vi "SutterController.vi"() -> ()   [LabVIEW 2014]
uses:
  SerialController/Serial Controller.lvclass
  GlobalVars.vi
  <vilib>/Analysis/Matrix/Numeric/Conversions/Array To Matrix - RA2.vi
  <vilib>/Analysis/Matrix/Numeric/Conversions/Array To Matrix - RA.vi
  <vilib>/Analysis/Matrix/Numeric/Multiply/Multiply - RM,RM.vi
  <vilib>/Analysis/Matrix/Numeric/Conversions/Matrix To Array - RM.vi
  <vilib>/Analysis/Matrix/NI_Matrix.lvlib
panel:
  in  "Feedback Gain":dbl=0.5 format="%#_13g"
  in  "AOD2Motor Coeff":dbl[][](array[numeric])=[[1.0473, -0.1243, -0.0724], [0.092, 0.9188, 0.1665], [-0.0112, -0.0078, 1.1755]]
  in  "Date Calibrated":string="3/2/2015"
  out "External_Z":dbl
  out "External_Y":dbl
  out "External_X":dbl
  in  "Perturb":bool
  in  "Perturb_Z":dbl
  in  "Perturb_Y":dbl
  in  "Perturb_X":dbl
  in  "Movement Refractory Period (sec)":dbl=1.0
  out "Last Movement Time":dbl
  out "PMEZ":dbl
  out "PMEY":dbl
  out "PMEX":dbl
  in  "Internal Movement Threshold":dbl=0.5 min=0.5 max=100.0 format="%#_13g"
  out "Communication Error":bool
  out "Over Cumulative Limit":bool
  in  "Max dZ":dbl=20.0 min=0.0 max=1000.0
  in  "Max dY":dbl=20.0 min=0.0 max=1000.0
  in  "Max dX":dbl=20.0 min=0.0 max=1000.0
  in  "Reset Cumulative Movements":bool
  out "Cumulative dZ":dbl
  out "Cumulative dY":dbl
  out "Cumulative dX":dbl
  in  "Standalone Operation":bool
  out "Reset":bool
  in  "Reset":bool
  in  "Simulated Tissue Movement":bool
  in  "External Movement Threshold":dbl=0.25 min=0.0 max=100.0 format="%#_13g"
  in  "Serial Port Share Friendly":bool
  in  "Tracking":bool
  out "Invalid Position":bool
  out "Current_Z":dbl
  out "Current_Y":dbl
  out "Current_X":dbl
  out "Loop Counter":i32
  in  "Set Position":bool
  in  "Position Source":bool=TRUE
  in  "Movement Speed":u16=3000 min=50 max=4000
  out "Current Position":dbl[](array[numeric])
  in  "stop":bool
  out "error out":errorcluster
  out "Moving":bool
  in  "Desired Position":dbl[](array[numeric])
  # "Off"
  # "On"
  # "Internal"
  # "External"
  # "Off"
  # "On"
  # "microns"
  # "Off"
  # "On"
  # "Desired Position"
  # "microns"
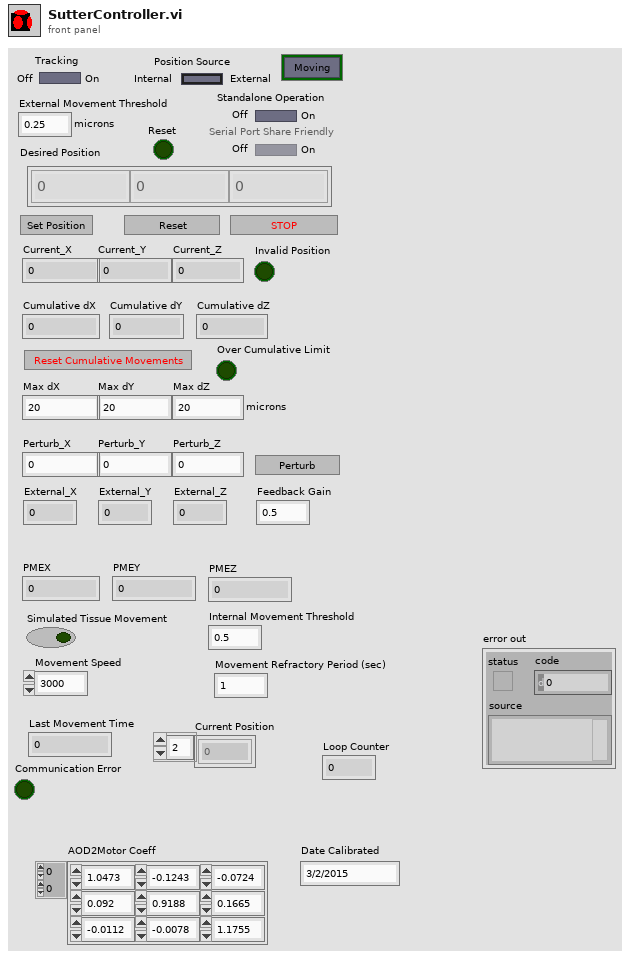
[diagram p1: front panel]
types:
  T1 = enum8{"Enabled", "Disabled", "Disabled and Grayed Out"}
  T2 = typedef "NI_Matrix.lvlib/RealMatrix.ctl" = dbl[][]
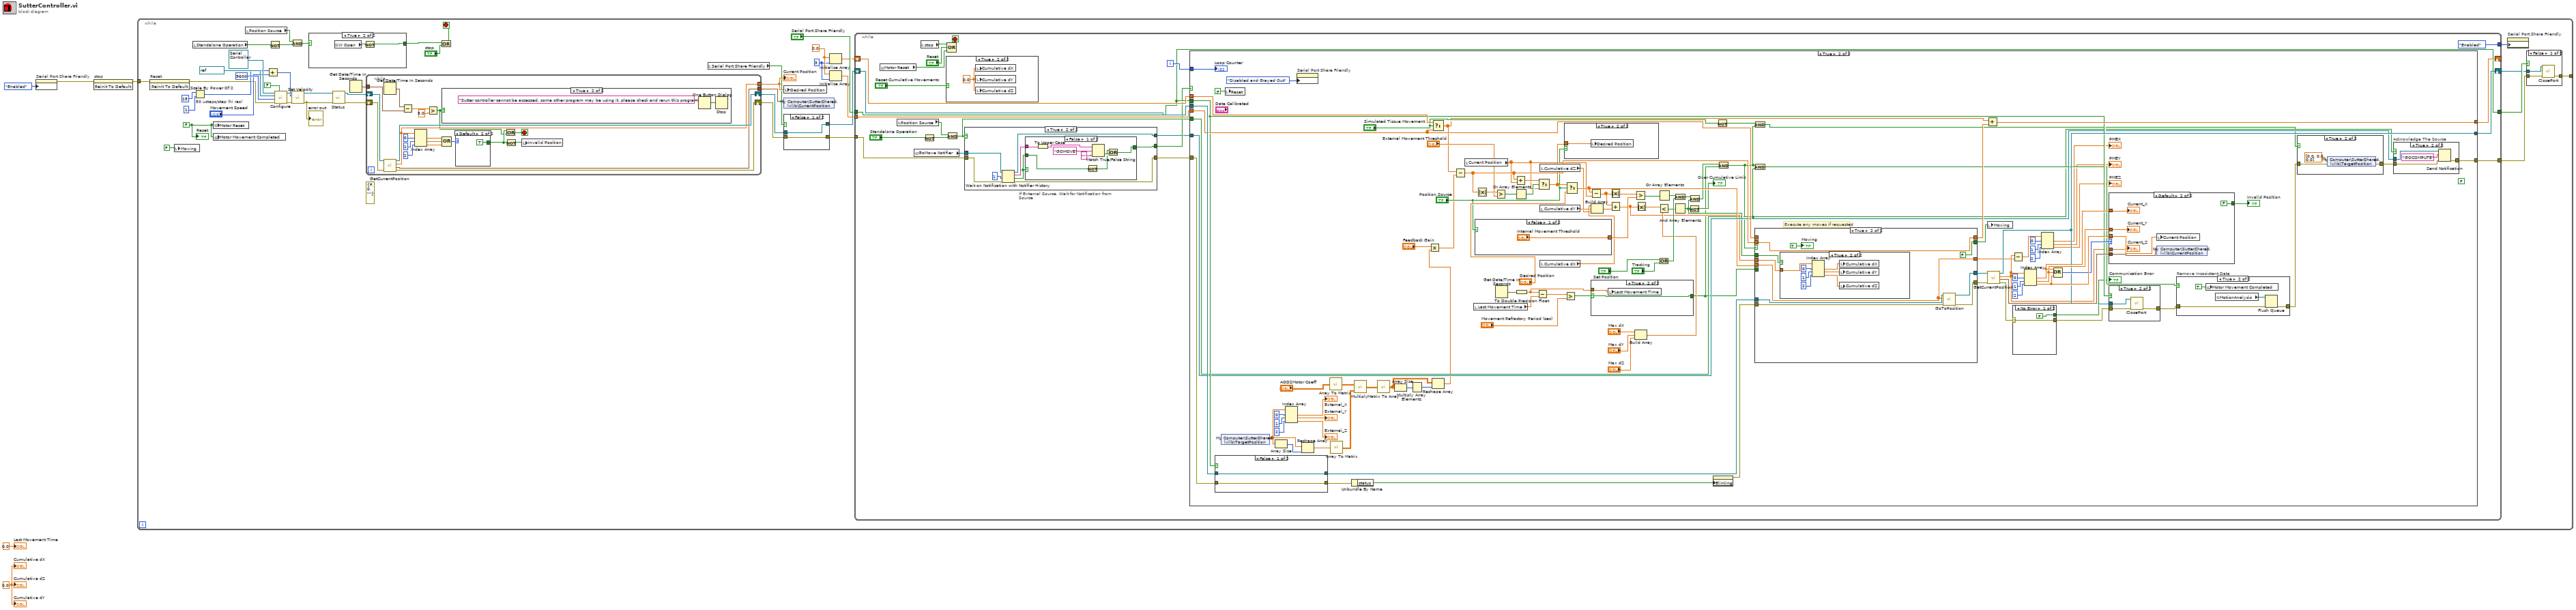
[diagram p0: block diagram]
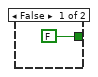
[diagram p2: hidden frame]
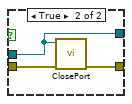
[diagram p4: hidden frame]
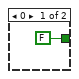
[diagram p6: hidden frame]
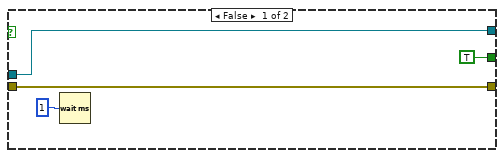
[diagram p8: hidden frame]
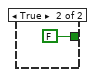
[diagram p9: hidden frame]
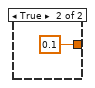
[diagram p13: hidden frame]
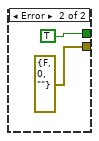
[diagram p14: hidden frame]
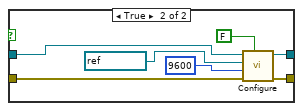
[diagram p19: hidden frame]
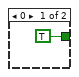
[diagram p20: hidden frame]
diagram:
  w3 = 0.0 ("Cumulative dX")
  n1 = property on="Serial Port Share Friendly" class="Bool (strict)"("DisabledEnum"=T1."Enabled" ("Disabled")) -> (error out=w4:errorcluster)  [unwired: 2 in, 1 out]
  n2 = invoke on="stop" class="Bool (strict)" method="Reinit To Default"(error in=w4) -> (error out=w2:errorcluster)  [unwired: 2 in, 2 out]
  n3 = while {
    tunnel: w2 -> [w21]
    tunnel: [w16] -> _
    stop <- w19 stop-if-true
    w6 = FALSE ("Reset")
    w26 = 3 ("dimension size")
    w27 = 0.0 ("element")
    (unwired) errorcluster {"status"=FALSE, "code"=0, "source"=""} ("error in (no error)")
    n4 = invoke on="Reset" class="Bool" method="Reinit To Default"(error in=w21) -> (error out=w22:errorcluster)  [unwired: 2 in, 2 out]
    n5 = local write "Moving"(FALSE ("Moving")) -> ()
    n6 = local read "Standalone Operation"() -> (w8:bool)
    n7 = Scale By Power Of 2 "50 usteps/step (hi res)"(n=i16 15, x=u16 1) -> (x*2^n=w39:u16)
    n8 = global write "GlobalVars.vi" "Motor Reset"(w6) -> ()
    n9 = global write "GlobalVars.vi" "Motor Movement Completed"(w6) -> ()
    n10 = local read "Position Source"() -> (w11:bool)
    n11 = Add(x=w39, y="Movement Speed") -> (x+y=w38:u16)
    n12 = Not(x=w8) -> (.not. x?=w10:bool)
    n13 = call-dynamic "Configure.vi"("Reset"=FALSE, "error in (no error)"=w22, "baud rate (9600)"=u32 9600, "VISA resource name"=refnum<visa-resource-name> "COM3", "Serial Controller in"=refnum<class "Serial Controller.lvclass"> refnum) -> ("error out"=w43:errorcluster, "Serial Controller out"=w44:refnum<class "Serial Controller.lvclass">)  [unwired: 5 in]
    n14 = And(x=w11, y=w10) -> (x .and. y?=w9:bool)
    n15 = call-dynamic "Set Velocity.vi"("error in (no error)"=w43, "Velocity"=w38, "Serial Controller in"=w44) -> ("error out"=w14:errorcluster, "Serial Controller out"=w15:refnum<class "Serial Controller.lvclass">)  [unwired: 7 in]
    "error out" <- w14
    n16 = case shown="True" w9 {
      tunnel: [FALSE w51] -> w18
      frame False {
      }
      frame True {
        n17 = global read "GlobalVars.vi" "VI Open"() -> (w52:bool)
        n18 = Not(x=w52) -> (.not. x?=w51:bool)
      }
    }
    n19 = call-dynamic "Status.vi"("Serial Controller in"=w15, "error in (no error)"=w14) -> ("Serial Controller out"=w13:refnum<class "Serial Controller.lvclass">, "error out"=w12:errorcluster)  [unwired: 5 in, 7 out]
    n20 = Get Date/Time In Seconds() -> (seconds since 1Jan1904=w7:timestamp)
    n21 = while {
      tunnel: [w79] -> w46
      tunnel: [w70] -> w36
      shift-right: [w80] -> w33
      shift-left: w13 -> [w78]
      shift-right: [w81] -> w35
      shift-left: w12 -> [w77]
      tunnel: w7 -> [w67]
      stop <- w63 stop-if-true
      n22 = Get Date/Time In Seconds() -> (seconds since 1Jan1904=w66:timestamp)
      n23 = call-dynamic "GetCurrentPosition.vi"("error in (no error)"=w77, "Serial Controller in"=w78) -> ("error out"=w81:errorcluster, "PositionBundle"=w79:cluster{"X":dbl, "Y":dbl, "Z":dbl, "Depth":dbl}, "Position"=w70:dbl[], "Serial Controller out"=w80:refnum<class "Serial Controller.lvclass">)  [unwired: 6 in]
      n24 = Subtract(x=w66, y=w67) -> (x-y=w65:dbl)
      n25 = Index Array(array=w70, index #1=0 ("index"), index #2=1 ("index"), index #3=2 ("index")) -> (element #1=w73:dbl, element #2=w72:dbl, element #3=w71:dbl)
      n26 = Greater?(x=w65, y=5.0) -> (0:w61:bool)
      n27 = case shown="True" w61 {
        frame False {
        }
        frame True {
          n28 = One Button Dialog(message="Sutter controller cannot be accessed, some other program may be using it, please check and rerun this program") -> (true=w82:bool)  [unwired: 1 in]
          n29 = Stop(stop? (T)=w82) -> ()
        }
      }
      n30 = Compound Arithmetic op=OR(w73, w72, w71) -> (w69:i32)
      n31 = case shown="Default" w69 {
        tunnel: [FALSE TRUE] -> w62
        frame 0 {
        }
        frame Default {
        }
      }
      n32 = Or(x=w62, y=w61) -> (x .or. y?=w63:bool)
      n33 = Not(x=w62) -> (.not. x?=w68:bool)
      n34 = local write "Invalid Position"(w68) -> ()
    }
    "Current Position" <- w36
    n35 = Or(x=w18, y="stop") -> (x .or. y?=w19:bool)
    n36 = local read "Serial Port Share Friendly"() -> (w32:bool)
    n37 = local write "Desired Position"(w36) -> ()
    n38 = shared-variable "My Computer\\SutterShared.lvlib\\CurrentPosition"(w46) -> ()  [unwired: 1 in, 1 out]
    n39 = case shown="False" w32 {
      tunnel: w35 -> [w57 w60]
      tunnel: [w57 w59] -> w34
      tunnel: w33 -> [w56 w58]
      tunnel: [w56 w58] -> w31
      frame False {
      }
      frame True {
        n40 = call-dynamic "ClosePort.vi"("error in (no error)"=w60, "Serial Controller in"=w58) -> ("error out"=w59:errorcluster)  [unwired: 9 in]
      }
    }
    n41 = Initialize Array(w27, w26) -> (w28:dbl[])
    n42 = Initialize Array(w27, w26) -> (w25:dbl[])
    n43 = while {
      shift-right: [w107] -> w23
      shift-left: w31 -> [w106]
      tunnel: w34 -> [w95]
      tunnel: "Serial Port Share Friendly" -> [w102]
      tunnel: [T1."Enabled" ("Disabled")] -> w29
      shift-right: [w105] -> _
      shift-left: w28 -> [w104]
      tunnel: w25 -> [w103]
      tunnel: [w102] -> w24
      tunnel: [w93] -> w17
      i -> [w108]
      stop <- w98 stop-if-true
      n44 = global read "GlobalVars.vi" "Motor Reset"() -> (w96:bool)
      n45 = local read "Position Source"() -> (w92:bool)
      n46 = global read "GlobalVars.vi" "GoMove Notifier"() -> (w86:refnum<notifier>)
      n47 = local read "stop"() -> (w100:bool)
      n48 = Not(x="Standalone Operation") -> (.not. x?=w90:bool)
      n49 = case shown="True" "Reset Cumulative Movements" {
        frame False {
        }
        frame True {
          w109 = 0.0 ("Cumulative dX")
          n50 = local write "Cumulative dX"(w109) -> ()
          n51 = local write "Cumulative dY"(w109) -> ()
          n52 = local write "Cumulative dZ"(w109) -> ()
        }
      }
      n53 = And(x=w92, y=w90) -> (x .and. y?=w89:bool)
      n54 = Compound Arithmetic op=OR(w100, "Reset", w96) -> (w98:bool)
      n55 = case "If External Source, Wait for Notification from Source" shown="True" w89 {
        tunnel: w95 -> [w113 w121]
        tunnel: [TRUE w117] -> w101
        tunnel: [w113 w120] -> w94
        tunnel: [w110 w115] -> w87
        tunnel: w86 -> [w110 w114]
        frame False {
          n56 = Wait (ms)(milliseconds to wait=u32 1) -> ()  [unwired: 1 out]
        }
        frame True {
          n57 = Wait on Notification with Notifier History(0:w114, 2:1 ("timeout in ms (-1)"), 3:w121) -> (8:w115:refnum<notifier>, 9:w118:string, 10:w116:bool, 11:w120:errorcluster)  [unwired: 1 in]
          n58 = case shown="False" w116 {
            tunnel: w118 -> [w129 _]
            tunnel: w116 -> [w124 _]
            tunnel: [w123 FALSE] -> w117
            frame False {
              n59 = To Upper Case(1:w129) -> (0:w128:string)
              n60 = Not(x=w124) -> (.not. x?=w125:bool)
              n61 = Match True/False String(2:"" ("false string"), 3:"GOMOVE" ("true string"), 4:w128) -> (0:w127:bool)  [unwired: 1 out]
              n62 = Or(x=w125, y=w127) -> (x .or. y?=w123:bool)
            }
            frame True {
            }
          }
        }
      }
      n63 = case shown="True" w101 {
        tunnel: w108 -> [_ w236]
        tunnel: [w132 w224] -> w107
        tunnel: w106 -> [w132 w220]
        tunnel: w94 -> [_ w218]
        tunnel: [w131 w209] -> w105
        tunnel: w104 -> [w131 w207]
        tunnel: w103 -> [_ w206]
        tunnel: w102 -> [_ w205]
        tunnel: [_ w202] -> w93
        tunnel: w87 -> [_ w201]
        tunnel: w89 -> [_ w176]
        frame False {
        }
        frame True {
          (unwired) FALSE
          # "Execute any moves if requested"
          n64 = case shown="False" w205 {
            tunnel: w220 -> [w272 w278]
            tunnel: [w272 w277] -> w219
            tunnel: w218 -> [w271 w275]
            tunnel: [w271 w274] -> w217
            frame False {
            }
            frame True {
              n65 = call-dynamic "Configure.vi"("Reset"=FALSE, "error in (no error)"=w275, "baud rate (9600)"=u32 9600, "VISA resource name"=refnum<visa-resource-name> "COM3", "Serial Controller in"=w278) -> ("error out"=w274:errorcluster, "Serial Controller out"=w277:refnum<class "Serial Controller.lvclass">)  [unwired: 5 in]
            }
          }
          n66 = shared-variable "My Computer\\SutterShared.lvlib\\TargetPosition"() -> (w139:dbl[])  [unwired: 1 in, 1 out]
          n67 = local write "Reset"(FALSE ("Ready")) -> ()
          n68 = Array Size(array=w139) -> (size(s)=w140:i32)
          n69 = Index Array(array=w139, index #1=0 ("index"), index #2=1 ("index"), index #3=2 ("index")) -> (element #1=→"External_X":dbl, element #2=→"External_Y":dbl, element #3=→"External_Z":dbl)
          n70 = property on="Serial Port Share Friendly" class="Bool (strict)"("DisabledEnum"=T1."Disabled and Grayed Out" ("Disabled")) -> ()  [unwired: 2 in, 2 out]
          n71 = Reshape Array(w139, w140) -> (w138:dbl[])
          n72 = call-poly <vilib>:"Array To Matrix.vi"("Real 2D Array"="AOD2Motor Coeff") -> ("Real Matrix"=w145:T2)
          n73 = call-poly <vilib>:"Array To Matrix.vi"("Real 1D Array"=w138) -> ("Real Matrix (Column Vector)"=w137:T2)
          n74 = Unbundle By Name(w217) -> ("status"=w243:bool)
          n75 = call-poly <vilib>:"Multiply.vi"("Real Matrix B"=w137, "Real Matrix A"=w145) -> ("A * B"=w144:T2)
          n76 = call-poly <vilib>:"Matrix To Array.vi"("Real Matrix"=w144) -> ("Real 2D Array"=w141:dbl[][])
          n77 = Array Size(array=w141) -> (size(s)=w143:i32[])
          n78 = Multiply Array Elements(1:w143) -> (0:w142:i32)
          n79 = Select(t=w207, s="Simulated Tissue Movement", f=w206) -> (s? t:f=w135:dbl[])
          n80 = Reshape Array(w141, w142) -> (w136:dbl[])
          n81 = Multiply(x="Feedback Gain", y=w136) -> (x*y=w134:dbl[])
          n82 = Subtract(x=w135, y=w134) -> (x-y=w204:dbl[])
          n83 = local read "Current Position"() -> (w198:dbl[])
          n84 = local read "Last Movement Time"() -> (w160:dbl)
          n85 = case shown="False" "Position Source" {
            tunnel: ["Internal Movement Threshold" 0.1 ("Tolerance for movement")] -> w240
            frame False {
            }
            frame True {
            }
          }
          n86 = Absolute Value(x=w204) -> (abs(x)=w213:dbl[])
          n87 = Greater?(x=w213, y="External Movement Threshold") -> (0:w216:bool[])
          n88 = Get Date/Time In Seconds() -> (seconds since 1Jan1904=w161:timestamp)
          n89 = Add(x=w204, y=w198) -> (x+y=w214:dbl[])
          n90 = Or Array Elements(Boolean array=w216) -> (logical OR=w215:bool)
          n91 = To Double Precision Float(number=w161) -> (double precision float=w156:dbl)
          n92 = Subtract(x=w156, y=w160) -> (x-y=w159:dbl)
          n93 = Select(t=w214, s=w215, f=w198) -> (s? t:f=w210:dbl[])
          n94 = local read "Cumulative dZ"() -> (w194:dbl)
          n95 = local read "Cumulative dY"() -> (w195:dbl)
          n96 = local read "Cumulative dX"() -> (w196:dbl)
          n97 = case shown="True" "Position Source" {
            tunnel: w210 -> [_ w266]
            frame False {
            }
            frame True {
              n98 = local write "Desired Position"(w266) -> ()
            }
          }
          n99 = Greater?(x=w159, y="Movement Refractory Period (sec)") -> (0:w157:bool)
          n100 = Select(t=w210, s="Position Source", f="Desired Position") -> (s? t:f=w197:dbl[])
          n101 = Subtract(x=w197, y=w198) -> (x-y=w177:dbl[])
          n102 = Build Array(w196, w195, w194) -> (w193:dbl[])
          n103 = case shown="True" w157 {
            selector: w157 -> [w244 w245]
            tunnel: w156 -> [_ w246]
            tunnel: [w244 w245] -> w153
            frame False {
            }
            frame True {
              n104 = local write "Last Movement Time"(w246) -> ()
            }
          }
          n105 = Absolute Value(x=w177) -> (abs(x)=w241:dbl[])
          n106 = Add(x=w177, y=w193) -> (x+y=w185:dbl[])
          n107 = Greater?(x=w241, y=w240) -> (0:w239:bool[])
          n108 = Build Array("Max dX", "Max dY", "Max dZ") -> (w192:dbl[])
          n109 = Absolute Value(x=w185) -> (abs(x)=w189:dbl[])
          n110 = Less?(x=w189, y=w192) -> (x < y?=w191:bool[])
          n111 = Or(x="Set Position", y="Tracking") -> (x .or. y?=w222:bool)
          n112 = Or Array Elements(Boolean array=w239) -> (logical OR=w179:bool)
          n113 = And(x=w179, y=w222) -> (x .and. y?=w190:bool)
          n114 = And Array Elements(Boolean array=w191) -> (logical AND=w183:bool)
          n115 = Not(x=w183) -> (.not. x?=→"Over Cumulative Limit":bool)
          n116 = And(x=w190, y=w183) -> (x .and. y?=w155:bool)
          n117 = property on="Desired Position" class="Arr (strict)"("Blinking"=w243) -> (error out=w238:errorcluster)  [unwired: 2 in, 1 out]
          n118 = Not(x="Simulated Tissue Movement") -> (.not. x?=w171:bool)
          n119 = And(x=w155, y=w153) -> (x .and. y?=w154:bool)
          n120 = And(x=w171, y=w154) -> (x .and. y?=w173:bool)
          n121 = And(x=w154, y=w176) -> (x .and. y?=w199:bool)
          n122 = case shown="True" w154 {
            tunnel: w219 -> [w293 w319]
            tunnel: [w292 w316] -> w234
            tunnel: w238 -> [w291 w318]
            tunnel: [w290 w315] -> w233
            tunnel: w197 -> [w294 w310]
            tunnel: [FALSE FALSE] -> w242
            tunnel: [w295 w313] -> w208
            tunnel: w206 -> [w295 _]
            tunnel: w204 -> [_ w313]
            tunnel: w185 -> [_ w312]
            tunnel: w183 -> [_ w311]
            tunnel: [w294 w310] -> w169
            tunnel: w153 -> [w287 _]
            frame False {
              n123 = And(x="Perturb", y=w287) -> (x .and. y?=w288:bool)
              n124 = case shown="True" w288 {
                tunnel: w293 -> [w298 w304]
                tunnel: [w298 w303] -> w292
                tunnel: w291 -> [w297 w302]
                tunnel: [w297 w301] -> w290
                frame False {
                }
                frame True {
                  n125 = local read "Current Position"() -> (w306:dbl[])
                  n126 = property on="Perturb" class="Bool (strict)"("Val(Sgnl)"=FALSE ("Value (Signaling)")) -> ()  [unwired: 2 in, 2 out]
                  n127 = Build Array("Perturb_X", "Perturb_Y", "Perturb_Z") -> (w305:dbl[])
                  n128 = Add(x=w306, y=w305) -> (x+y=w300:dbl[])
                  n129 = call-dynamic "GoToPosition.vi"("error in (no error)"=w302, "Position"=w300, "Serial Controller in"=w304) -> ("error out"=w301:errorcluster, "Serial Controller out"=w303:refnum<class "Serial Controller.lvclass">)  [unwired: 6 in, 1 out]
                }
              }
            }
            frame True {
              n130 = case shown="True" w311 {
                tunnel: w312 -> [_ w326]
                frame False {
                }
                frame True {
                  n131 = Index Array(array=w326, index #1=0 ("index"), index #2=1 ("index"), index #3=2 ("index")) -> (element #1=w322:dbl, element #2=w321:dbl, element #3=w320:dbl)
                  n132 = local write "Cumulative dX"(w322) -> ()
                  n133 = local write "Cumulative dY"(w321) -> ()
                  n134 = local write "Cumulative dZ"(w320) -> ()
                }
              }
              n135 = call-dynamic "GoToPosition.vi"("error in (no error)"=w318, "Position"=w310, "Serial Controller in"=w319) -> ("error out"=w315:errorcluster, "Serial Controller out"=w316:refnum<class "Serial Controller.lvclass">)  [unwired: 6 in, 1 out]
              "Moving" <- TRUE ("Boolean")
            }
          }
          n136 = Add(x=w135, y=w208) -> (x+y=w209:dbl[])
          n137 = local write "Moving"(w242) -> ()
          n138 = call-dynamic "GetCurrentPosition.vi"("error in (no error)"=w233, "Serial Controller in"=w234) -> ("error out"=w182:errorcluster, "PositionBundle"=w235:cluster{"X":dbl, "Y":dbl, "Z":dbl, "Depth":dbl}, "Position"=w170:dbl[], "Serial Controller out"=w224:refnum<class "Serial Controller.lvclass">)  [unwired: 6 in]
          n139 = Subtract(x=w170, y=w169) -> (x-y=w168:dbl[])
          n140 = case shown="No Error" w182 {
            selector: w182 -> [w252 _]
            tunnel: [w252 errorcluster {"status"=FALSE, "code"=0, "source"=""} ("error out")] -> w181
            tunnel: [FALSE ("Communication Error") TRUE ("Communication Error")] -> w180
            frame No Error {
            }
            frame Error {
            }
          }
          "Communication Error" <- w180
          n141 = Index Array(array=w170, index #1=0 ("index"), index #2=1 ("index"), index #3=2 ("index")) -> (element #1=w229:dbl, element #2=w228:dbl, element #3=w227:dbl)
          n142 = Index Array(array=w168, index #1=0 ("index"), index #2=1 ("index"), index #3=2 ("index")) -> (element #1=→"PMEX":dbl, element #2=→"PMEY":dbl, element #3=→"PMEZ":dbl)
          n143 = Compound Arithmetic op=OR(w229, w228, w227) -> (w226:i32)
          n144 = case shown="Default" w226 {
            tunnel: w235 -> [_ w286]
            tunnel: w227 -> [_ w285]
            tunnel: w228 -> [_ w284]
            tunnel: w229 -> [_ w283]
            tunnel: w170 -> [_ w282]
            tunnel: [TRUE FALSE] -> w225
            frame 0 {
            }
            frame Default {
              n145 = local write "Current Position"(w282) -> ()
              n146 = shared-variable "My Computer\\SutterShared.lvlib\\CurrentPosition"(w286) -> ()  [unwired: 1 in, 1 out]
              "Current_X" <- w283
              "Current_Y" <- w284
              "Current_Z" <- w285
            }
          }
          "Invalid Position" <- w225
          n147 = case shown="True" w205 {
            tunnel: w224 -> [_ w270]
            tunnel: w181 -> [w267 w269]
            tunnel: [w267 w268] -> w200
            frame False {
            }
            frame True {
              n148 = call-dynamic "ClosePort.vi"("error in (no error)"=w269, "Serial Controller in"=w270) -> ("error out"=w268:errorcluster)  [unwired: 9 in]
            }
          }
          n149 = case "Remove Incosistent Data" shown="True" w199 {
            tunnel: w200 -> [w256 w260]
            tunnel: [w256 w259] -> w175
            frame False {
            }
            frame True {
              n150 = global write "GlobalVars.vi" "Motor Movement Completed"(TRUE ("Motor Movement Completed")) -> ()
              n151 = global read "GlobalVars.vi" "MotionAnalysis"() -> (w258:refnum<queue>)
              n152 = Flush Queue(queue=w258, error in (no error)=w260) -> (error out=w259:errorcluster)  [unwired: 2 out]
            }
          }
          n153 = case shown="True" w173 {
            tunnel: w175 -> [_ w248]
            tunnel: [_ w247] -> w174
            frame False {
            }
            frame True {
              n154 = shared-variable "My Computer\\SutterShared.lvlib\\TargetPosition"(dbl[] [0.0, 0.0, 0.0] ("TargetPosition"), error in=w248) -> (error out=w247:errorcluster)
            }
          }
          n155 = case "Acknowledge The Source" shown="True" w176 {
            tunnel: w174 -> [w261 w262]
            tunnel: [w261 w265] -> w202
            tunnel: w201 -> [_ w263]
            frame False {
            }
            frame True {
              n156 = Send Notification(notification="GOCOMPUTE", notifier=w263, error in (no error)=w262) -> (error out=w265:errorcluster)  [unwired: 1 out]
            }
          }
          "Loop Counter" <- w236
        }
      }
    }
    n157 = property on="Serial Port Share Friendly" class="Bool (strict)"("DisabledEnum"=w29) -> ()  [unwired: 2 in, 2 out]
    n158 = case shown="False" w24 {
      tunnel: w23 -> [w55 _]
      tunnel: w17 -> [w54 _]
      tunnel: [w53 _] -> w16
      frame False {
        n159 = call-dynamic "ClosePort.vi"("error in (no error)"=w54, "Serial Controller in"=w55) -> ("error out"=w53:errorcluster)  [unwired: 9 in]
      }
      frame True {
      }
    }
    "Reset" <- w6
  }
  "Cumulative dX" <- w3
  "Cumulative dY" <- w3
  "Cumulative dZ" <- w3
  "Last Movement Time" <- 0.0 ("Last Movement Time")
